vi "Do Core.vi"(8 "error in":errorcluster, 9 "Actor in":refnum<class "Actor.lvclass">, 11 "Reply Message":refnum<class "Reply Msg Msg.lvclass">) -> (0 "error out":errorcluster, 1 "Actor out":refnum<class "Actor.lvclass">, 2 "Reply":variant)   [LabVIEW 2023, in "Target Reply Time Test Actor.lvlib" / "Reply Msg Msg.lvclass"]
doc: "(<B>Filename</B>: Actor Framework.lvlib:Reply Msg.lvclass:Do Core.vi)\n\nDefines what an actor does when it receives <B>Reply Message</B>. This method also defines the <B>Reply</B> that is returned to the actor that sent <B>Reply Message</B>.\n\nBy default, this method does nothing, and <B>Reply</B> is the ancestor Message class. A child class must override this method to define behavior and specify a child of the Message class to return in the <B>Reply</B> output."
uses:
  Reply Msg Msg.lvclass
  <vilib>/ActorFramework/Actor/Actor.lvclass
  Target Reply Time Test Actor/Target Reply Time Test Actor.lvclass
  Reply Msg Msg.lvclass/Reply Msg Msg.ctl
  a3c53ac0-5788-4fdb-8af4-53e1f014a370.vi
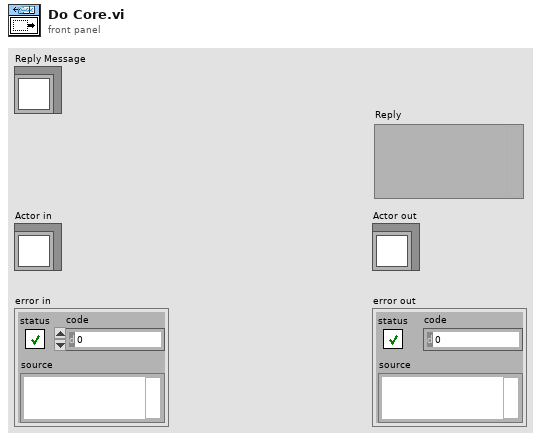
[diagram p1: front panel]
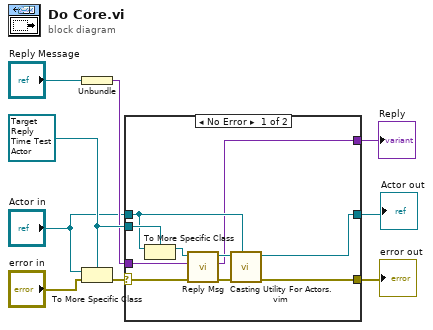
[diagram p0: block diagram]
diagram:
  w8 = refnum<class "Target Reply Time Test Actor.lvclass"> refnum ("Actor in")
  n1 = Unbundle("Reply Message") -> (w7:variant)
  n2 = To More Specific Class(target class=w8, reference="Actor in", error in="error in") -> (error out=w9:errorcluster)  [unwired: 1 out]
  n3 = case shown="No Error" w9 {
    selector: w9 -> [w19 w21]
    tunnel: [w13 w21] -> w3
    tunnel: [w14 w20] -> w2
    tunnel: "Actor in" -> [w16 w20]
    tunnel: w8 -> [w17 _]
    tunnel: w7 -> [w11 _]
    tunnel: [w10 _] -> w1
    frame No Error {
      n4 = To More Specific Class(target class=w17, reference=w16) -> (specific class reference=w18:refnum<class "Target Reply Time Test Actor.lvclass">)  [unwired: 1 in, 1 out]
      n5 = call-dynamic "Reply Msg.vi"("error in"=w19, "Input"=w11, "Target Reply Time Test Actor in"=w18) -> ("error out"=w12:errorcluster, "Output"=w10:variant, "Target Reply Time Test Actor out"=w15:refnum<class "Target Reply Time Test Actor.lvclass">)  [unwired: 6 in]
      n6 = call "Casting Utility For Actors.vim"("type"=w16, "error in (no error)"=w12, "Actor in"=w15) -> ("error out"=w13:errorcluster, "Actor out"=w14:refnum<class "Actor.lvclass">)  [unwired: 7 in]
    }
    frame Error {
      # "If type check fails, pass the original object out again."
    }
  }
  "error out" <- w3
  "Actor out" <- w2
  "Reply" <- w1
